vi "Display Info.vi"(7 "Layout ref":refnum<vi>, 8 "error in (no error)":errorcluster, 9 "Modify (F) /Add [T]":bool, 10 "Names in use":string[](array[string]), 11 "NI Card in":refnum<class "NI Card.lvclass">=refnum) -> (0 "error out":errorcluster, 1 "Names in use out":string[](array[string]), 2 "Changes Made?":bool=TRUE, 3 "NI Card out":refnum<class "NI Card.lvclass">)   [LabVIEW 2013, in "NI Card.lvclass"]
uses:
  NI Card.lvclass
  TypeDefs/ColumnAppearCluster.ctl
  TypeDefs/DigitalColumnAppearCluster.ctl
  ColumnVIs/DigitalCol/DigitalCol.lvclass
  ColumnVIs/Column/Column.lvclass
  NI Card.lvclass/NI Card.ctl
panel:
  in  "Set All Analogs":T1={"Column Name"="", "Width"=30, "Bkgd"=[16448250], "Text"=[0]}
  in  "Set All Digitals":T2={"Column Name"="", "Width"=15, "Bkgd"=[1985280, 6618880, 14090026], "Text"=[16448250, 0, 0]}
  in  "Terminal Info":T3={"Trigger terminal"="", "Master\nTrigger Line"=23, "Trigger Mirror"="", "AO Lines"=0, "DO Channel"="", "DO Lines"=0, "AI Pause Line"="", "AI Sample Rate"=0.0, "AI Lines"=0}
  in  "Analog Input Channels":T4(array[cluster])
  in  "Analog Output Channels":T5(array[cluster])
  in  "Digital Output Channels":T2[](array[typedef])
  in  "Cancel":bool
  in  "Done":bool
  in  "Device Description":string
  in  "Name":string="ni"
  # "All Selected channels MUST be from same device! Same goes for \"Terminal Info.\""
  # "Trace color currently does nothing."
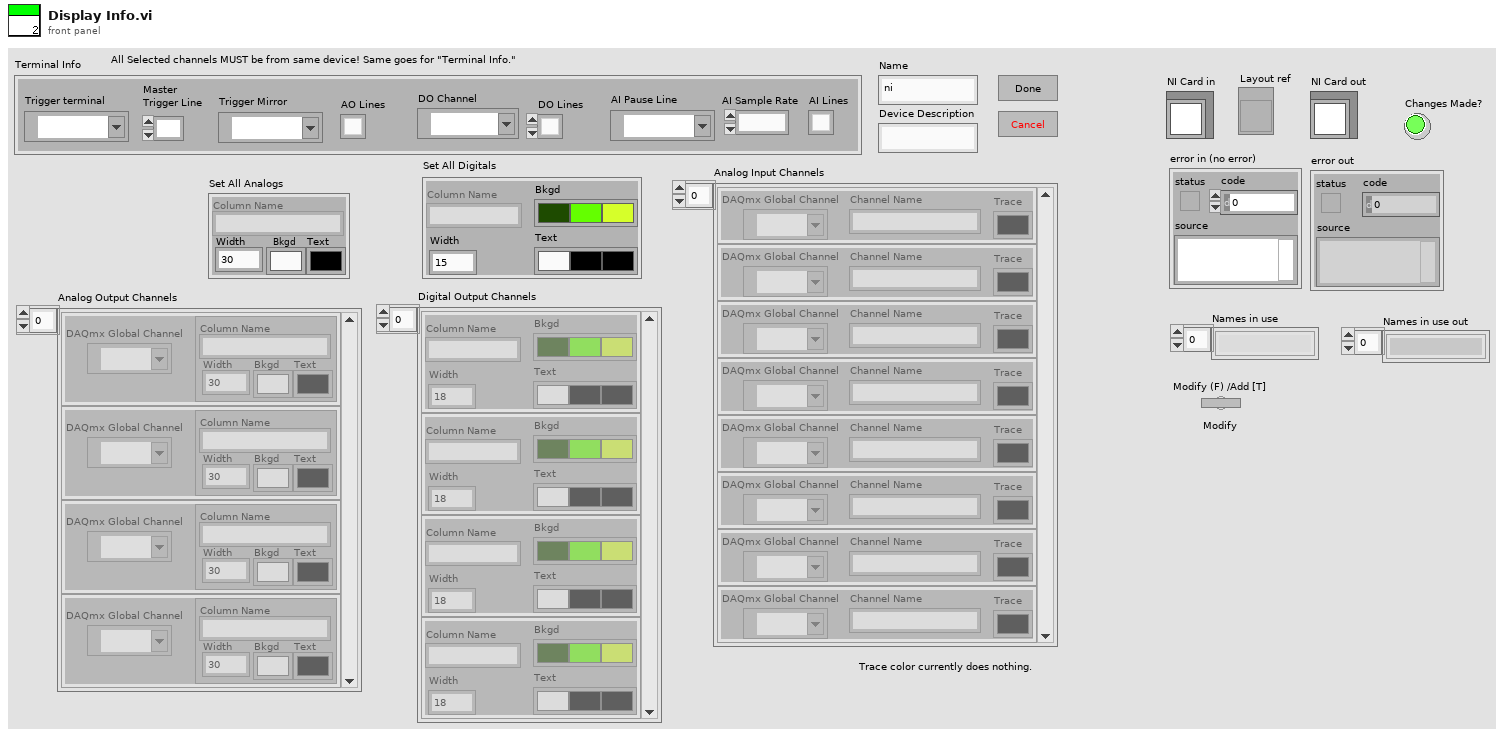
[diagram p1: front panel]
types:
  T1 = typedef "ColumnAppearCluster.ctl" = cluster{"Column Name":string, "Width":u32, "Bkgd":u32[], "Text":u32[]}
  T2 = typedef "DigitalColumnAppearCluster.ctl" = cluster{"Column Name":string, "Width":u32, "Bkgd":u32[], "Text":u32[]}
  T3 = cluster{"Trigger terminal":tag, "Master\nTrigger Line":u16, "Trigger Mirror":tag, "AO Lines":i32, "DO Channel":refnum<k21>, "DO Lines":i32, "AI Pause Line":tag, "AI Sample Rate":dbl, "AI Lines":i32}
  T4 = cluster{"DAQmx Global Channel":refnum<k21>, "Channel Name":string, "Trace":u32[]}[]
  T5 = cluster{"Column Appearance":T1, "DAQmx Global Channel":refnum<k21>}[]
  T6 = cluster{"AI Pause Line":tag, "AI Sample Rate":dbl, "Trigger terminal":tag, "DO Channel":refnum<k21>, "Trigger Mirror":tag}
  T7 = cluster{"DAQmx Global Channel":refnum<k21>, "String":string}[]
  T8 = cluster{"DAQmx Global Channel":refnum<k21>, "Channel Name":string, "Trace":u32[]}
  T9 = cluster{"Column Appearance":T1, "DAQmx Global Channel":refnum<k21>}
  T10 = cluster{"DAQmx Global Channel":refnum<k21>, "Column Name":string}
  T11 = cluster{"DAQmx Global Channel":refnum<k21>, "Channel Name":string}
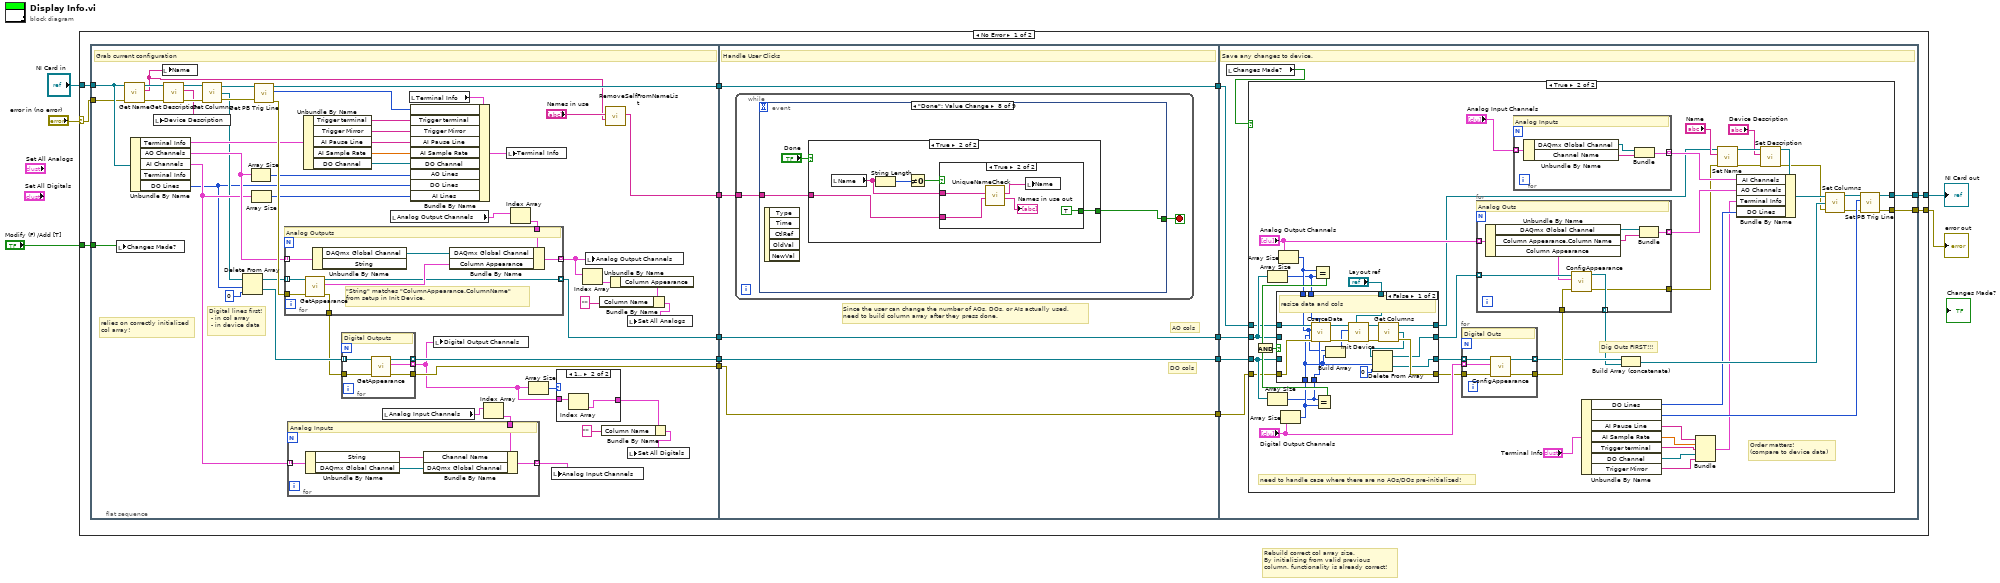
[diagram p0: block diagram]
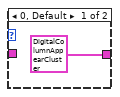
[diagram p2: hidden frame]
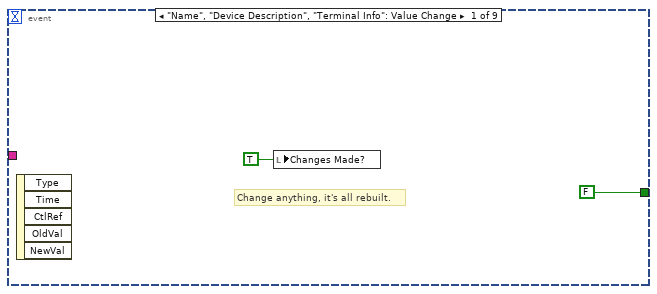
[diagram p3: hidden frame]
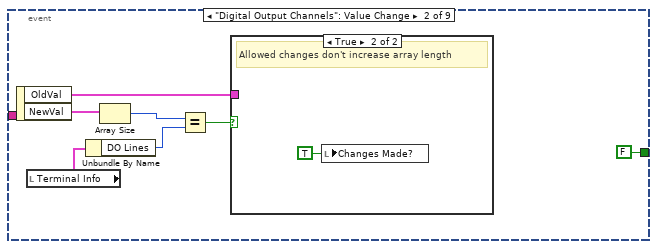
[diagram p4: hidden frame]
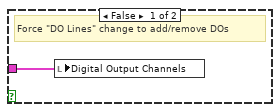
[diagram p5: hidden frame]
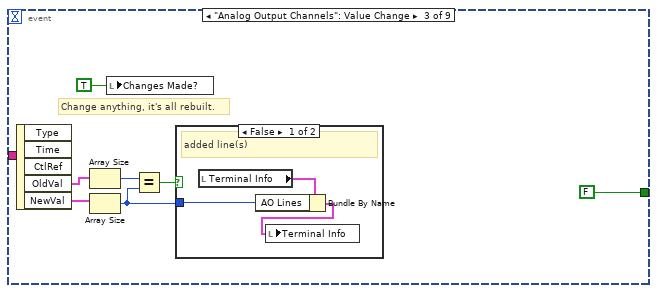
[diagram p6: hidden frame]
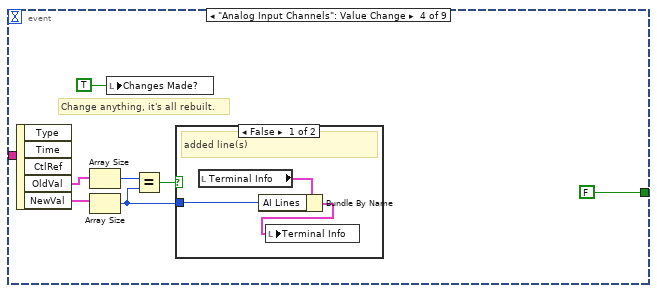
[diagram p8: hidden frame]
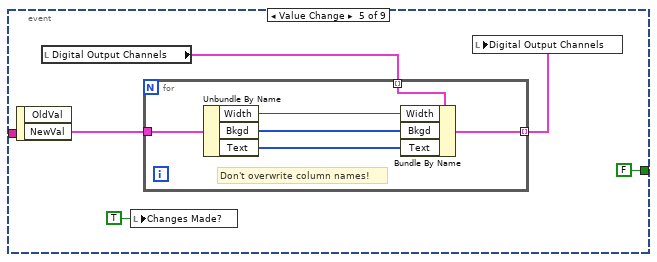
[diagram p10: hidden frame]
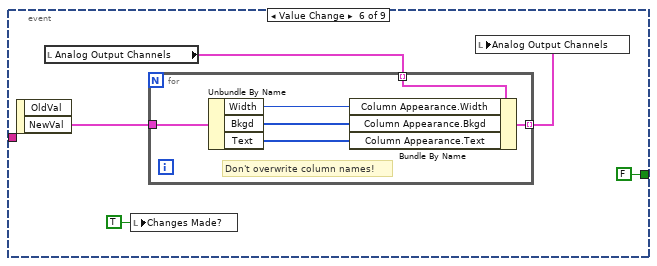
[diagram p11: hidden frame]
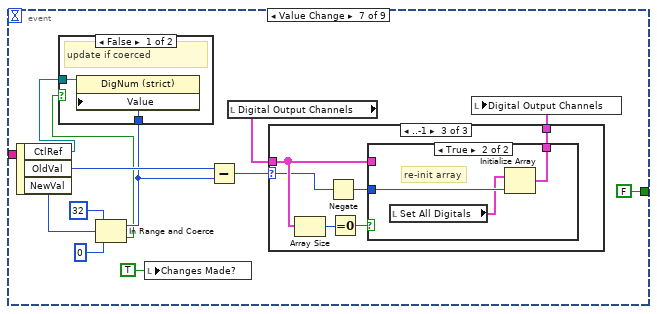
[diagram p12: hidden frame]
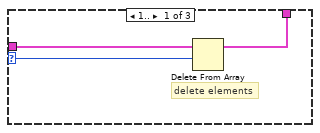
[diagram p14: hidden frame]
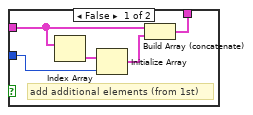
[diagram p16: hidden frame]
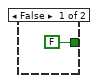
[diagram p17: hidden frame]
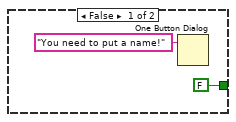
[diagram p18: hidden frame]
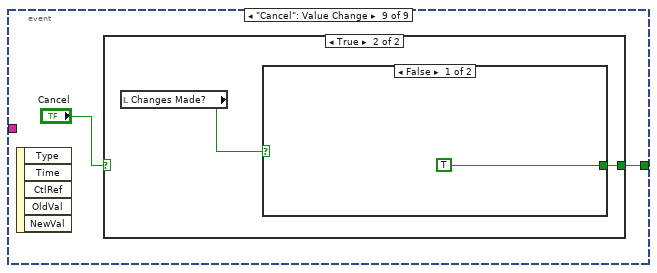
[diagram p19: hidden frame]
diagram:
  # "Rebuild correct col array size.\nBy initializing from valid previous\ncolumn, functionality is already correct!"
  n1 = case shown="No Error" "error in (no error)" {
    selector: "error in (no error)" -> [w16 w308]
    tunnel: "NI Card in" -> [w19 w309]
    tunnel: [w9 w309] -> w3
    tunnel: [w8 w308] -> w2
    tunnel: "Modify (F) /Add [T]" -> [w7 _]
    frame No Error {
      n2 = flat-sequence {
        tunnel: w19 -> [w69]
        tunnel: [w64] -> w18
        tunnel: w16 -> [w43]
        tunnel: [w42] -> w15
        tunnel: [w41] -> w14
        tunnel: [w40] -> w13
        tunnel: w7 -> [w23]
        tunnel: [w20] -> w6
        tunnel: w18 -> [w98]
        tunnel: [w98] -> w17
        tunnel: w15 -> [w95]
        tunnel: w14 -> [w96]
        tunnel: w13 -> [w97]
        tunnel: [w97] -> w12
        tunnel: [w96] -> w11
        tunnel: [w95] -> w10
        tunnel: w6 -> [w94]
        tunnel: w17 -> [w216]
        tunnel: w12 -> [w218]
        tunnel: w11 -> [w217]
        tunnel: w10 -> [w213]
        tunnel: [w215] -> w9
        tunnel: [w214] -> w8
        frame #0 {
          # "relies on correctly initialized\ncol array!"
          # "Digital lines first!\n - in col array\n - in device data"
          # "Grab current configuration"
          n3 = local write "Changes Made?"(w23) -> ()
          n4 = call-dynamic "Get Name.vi"("error in (no error)"=w43, "Device in"=w69) -> ("error out"=w68:errorcluster, "Name"=w21:string, "Device out"=w70:refnum<class "NI Card.lvclass">)  [unwired: 7 in]
          n5 = Unbundle By Name(w69) -> ("Terminal Info"=w57:T6, "AO Channels"=w53:T7, "AI Channels"=w52:T7, "DO Lines"=w32:i32)  [unwired: 1 out]
          n6 = local write "Name"(w21) -> ()
          n7 = call-dynamic "Get Description.vi"("error in (no error)"=w68, "Device in"=w70) -> ("error out"=w66:errorcluster, "Device Description"=w51:string, "Device out"=w67:refnum<class "NI Card.lvclass">)  [unwired: 7 in]
          n8 = local write "Device Description"(w51) -> ()
          n9 = call-dynamic "Get Columns.vi"("Device in"=w67, "error in (no error)"=w66) -> ("Device out"=w65:refnum<class "NI Card.lvclass">, "Columns"=w50:refnum<class "Column.lvclass">[], "error out"=w63:errorcluster)
          n10 = Delete From Array(array=w50, length=w32, index=0) -> (deleted portion=w47:refnum<class "Column.lvclass">[], array with subset deleted=w48:refnum<class "Column.lvclass">[])
          n11 = Array Size(array=w53) -> (size(s)=w55:i32)
          n12 = Array Size(array=w52) -> (size(s)=w54:i32)
          n13 = call-dynamic "Get PB Trig Line.vi"("error in (no error)"=w63, "Device in"=w65) -> ("error out"=w71:errorcluster, "PB Trigger Line"=w45:u16, "Device out"=w64:refnum<class "NI Card.lvclass">)  [unwired: 7 in]
          n14 = Unbundle By Name(w57) -> ("Trigger terminal"=w61:tag, "Trigger Mirror"=w62:tag, "AI Pause Line"=w60:tag, "AI Sample Rate"=w59:dbl, "DO Channel"=w58:refnum<k21>)
          n15 = local read "Analog Input Channels"() -> (w36:T4)
          n16 = local read "Analog Output Channels"() -> (w38:T5)
          n17 = local read "Terminal Info"() -> (w39:T3)
          n18 = Bundle By Name(cluster=w39, "Master\nTrigger Line"=w45, "Trigger terminal"=w61, "Trigger Mirror"=w62, "AI Pause Line"=w60, "AI Sample Rate"=w59, "DO Channel"=w58, "AO Lines"=w55, "DO Lines"=w32, "AI Lines"=w54) -> (w56:T3)
          n19 = Index Array(array=w36) -> (element=w35:T8)  [unwired: 1 in]
          n20 = for {
            tunnel: w52 -> [w84] mode=indexing
            tunnel: w35 -> [w83]
            tunnel: [w80] -> w46 mode=indexing
            # "Analog Inputs"
            n21 = Unbundle By Name(w84) -> ("String"=w82:string, "DAQmx Global Channel"=w81:refnum<k21>)
            n22 = Bundle By Name(cluster=w83, "Channel Name"=w82, "DAQmx Global Channel"=w81) -> (w80:T8)
          }
          n23 = local write "Terminal Info"(w56) -> ()
          n24 = Index Array(array=w38) -> (element=w37:T9)  [unwired: 1 in]
          n25 = for {
            tunnel: w53 -> [w93] mode=indexing
            tunnel: w48 -> [w89] mode=indexing
            tunnel: [w90] -> w34 mode=indexing
            tunnel: w71 -> [w88]
            tunnel: [w87] -> w44
            tunnel: [w86] -> w40 mode=indexing
            tunnel: w37 -> [w85]
            # "\"String\" matches \"ColumnAppearance.ColumnName\"\nfrom setup in Init Device."
            # "Analog Outputs"
            n26 = call "GetAppearance.vi"("error in (no error)"=w88, "Column in"=w89) -> ("error out"=w87:errorcluster, "Column Appearance"=w91:T1, "Column out"=w86:refnum<class "Column.lvclass">)  [unwired: 7 in]
            n27 = Unbundle By Name(w93) -> ("DAQmx Global Channel"=w92:refnum<k21>)  [unwired: 1 out]
            n28 = Bundle By Name(cluster=w85, "DAQmx Global Channel"=w92, "Column Appearance"=w91) -> (w90:T9)
          }
          n29 = for {
            tunnel: w47 -> [w79] mode=indexing
            tunnel: [w78] -> w31 mode=indexing
            tunnel: w44 -> [w77]
            tunnel: [w76] -> w42
            tunnel: [w75] -> w41 mode=indexing
            # "Digital Outputs"
            n30 = call "GetAppearance.vi"("error in (no error)"=w77, "Column in"=w79) -> ("error out"=w76:errorcluster, "Column Appearance"=w78:T1, "Column out"=w75:refnum<class "Column.lvclass">)  [unwired: 7 in]
          }
          n31 = local write "Digital Output Channels"(w31) -> ()
          n32 = Array Size(array=w31) -> (size(s)=w30:i32)
          n33 = local write "Analog Input Channels"(w46) -> ()
          n34 = case shown="1.." w30 {
            tunnel: w31 -> [_ w74]
            tunnel: [T2 {"Column Name"="", "Width"=15, "Bkgd"=[1985280, 6618880, 14090026], "Text"=[16448250, 0, 0]} ("Set All Digitals") w73] -> w25
            frame 0, Default {
            }
            frame 1.. {
              n35 = Index Array(array=w74) -> (element=w73:T1)  [unwired: 1 in]
            }
          }
          n36 = Index Array(array=w34) -> (element=w33:T9)  [unwired: 1 in]
          n37 = local write "Analog Output Channels"(w34) -> ()
          n38 = Bundle By Name(cluster=w25, "Column Name"="") -> (w24:T1)
          n39 = call "RemoveSelfFromNameList.vi"("self Name"=w21, "Names in use"="Names in use") -> ("Reserved Names"=w20:string[])  [unwired: 9 in]
          n40 = Unbundle By Name(w33) -> ("Column Appearance"=w29:T1)
          n41 = Bundle By Name(cluster=w29, "Column Name"="") -> (w27:T1)
          n42 = local write "Set All Analogs"(w27) -> ()
          n43 = local write "Set All Digitals"(w24) -> ()
        }
        frame #1 {
          # "DO cols"
          # "AO cols"
          # "Since the user can change the number of AOs, DOs, or AIs actually used, \nneed to build column array after they press done."
          # "Handle User Clicks"
          n44 = while {
            tunnel: w94 -> [w99]
            stop <- w100 stop-if-true
            n45 = event shown="[7] \"Done\": Value Change" {
              selector: _ -> [_ _ _ _ _ _ _ _ _]
              dyn-events: _ -> [_ _ _ _ _ _ _ _ _]
              timeout: _ -> [_ _ _ _ _ _ _ _ _]
              tunnel: [FALSE ("T button?") FALSE ("T button?") FALSE ("T button?") FALSE ("T button?") FALSE ("T button?") FALSE ("T button?") FALSE ("T button?") w187 w202] -> w100
              tunnel: w99 -> [_ _ _ _ _ _ _ w186 _]
              event "Name", "Device Description", "Terminal Info": Value Change {
                # "Change anything, it's all rebuilt."
                n46 = event-data() -> ()  [unwired: 1 in, 5 out]
                n47 = local write "Changes Made?"(TRUE) -> ()
              }
              event "Digital Output Channels": Value Change {
                n48 = event-data() -> ("OldVal"=w104:T2[], "NewVal"=w109:T2[])  [unwired: 1 in]
                n49 = local read "Terminal Info"() -> (w108:T3)
                n50 = Unbundle By Name(w108) -> ("DO Lines"=w106:i32)
                n51 = Array Size(array=w109) -> (size(s)=w107:i32)
                n52 = Equal?(x=w107, y=w106) -> (x = y?=w105:bool)
                n53 = case shown="True" w105 {
                  tunnel: w104 -> [w110 _]
                  frame False {
                    # "Force \"DO Lines\" change to add/remove DOs"
                    n54 = local write "Digital Output Channels"(w110) -> ()
                  }
                  frame True {
                    # "Allowed changes don't increase array length"
                    n55 = local write "Changes Made?"(TRUE ("Changes Made?")) -> ()
                  }
                }
              }
              event "Analog Output Channels": Value Change {
                # "Change anything, it's all rebuilt."
                n56 = event-data() -> ("OldVal"=w115:T5, "NewVal"=w116:T5)  [unwired: 1 in, 3 out]
                n57 = Array Size(array=w115) -> (size(s)=w114:i32)
                n58 = Array Size(array=w116) -> (size(s)=w112:i32)
                n59 = local write "Changes Made?"(TRUE) -> ()
                n60 = Equal?(x=w114, y=w112) -> (x = y?=w113:bool)
                n61 = case shown="False" w113 {
                  tunnel: w112 -> [w120 _]
                  frame False {
                    # "added line(s)"
                    n62 = local read "Terminal Info"() -> (w121:T3)
                    n63 = Bundle By Name(cluster=w121, "AO Lines"=w120) -> (w119:T3)
                    n64 = local write "Terminal Info"(w119) -> ()
                  }
                  frame True {
                    # "same number of lines"
                  }
                }
              }
              event "Analog Input Channels": Value Change {
                # "Change anything, it's all rebuilt."
                n65 = event-data() -> ("OldVal"=w125:T4, "NewVal"=w126:T4)  [unwired: 1 in, 3 out]
                n66 = Array Size(array=w125) -> (size(s)=w124:i32)
                n67 = Array Size(array=w126) -> (size(s)=w122:i32)
                n68 = local write "Changes Made?"(TRUE) -> ()
                n69 = Equal?(x=w124, y=w122) -> (x = y?=w123:bool)
                n70 = case shown="False" w123 {
                  tunnel: w122 -> [w130 _]
                  frame False {
                    # "added line(s)"
                    n71 = local read "Terminal Info"() -> (w131:T3)
                    n72 = Bundle By Name(cluster=w131, "AI Lines"=w130) -> (w129:T3)
                    n73 = local write "Terminal Info"(w129) -> ()
                  }
                  frame True {
                    # "same number of lines"
                  }
                }
              }
              event Value Change {
                n74 = event-data() -> ("NewVal"=w132:T2)  [unwired: 1 in, 1 out]
                n75 = local read "Digital Output Channels"() -> (w134:T2[])
                n76 = local write "Changes Made?"(TRUE ("Changes Made?")) -> ()
                n77 = for {
                  tunnel: w134 -> [w142] mode=indexing
                  tunnel: [w141] -> w133 mode=indexing
                  tunnel: w132 -> [w140]
                  # "Don't overwrite column names!"
                  n78 = Unbundle By Name(w140) -> ("Width"=w139:u32, "Bkgd"=w138:u32[], "Text"=w137:u32[])
                  n79 = Bundle By Name(cluster=w142, "Width"=w139, "Bkgd"=w138, "Text"=w137) -> (w141:T2)
                }
                n80 = local write "Digital Output Channels"(w133) -> ()
              }
              event Value Change {
                n81 = event-data() -> ("NewVal"=w143:T1)  [unwired: 1 in, 1 out]
                n82 = local read "Analog Output Channels"() -> (w145:T5)
                n83 = local write "Changes Made?"(TRUE ("Changes Made?")) -> ()
                n84 = for {
                  tunnel: w145 -> [w153] mode=indexing
                  tunnel: [w152] -> w144 mode=indexing
                  tunnel: w143 -> [w151]
                  # "Don't overwrite column names!"
                  n85 = Unbundle By Name(w151) -> ("Width"=w150:u32, "Bkgd"=w149:u32[], "Text"=w148:u32[])
                  n86 = Bundle By Name(cluster=w153, "Column Appearance.Width"=w150, "Column Appearance.Bkgd"=w149, "Column Appearance.Text"=w148) -> (w152:T9)
                }
                n87 = local write "Analog Output Channels"(w144) -> ()
              }
              event "Terminal Info.DO Lines": Value Change {
                n88 = event-data() -> ("CtlRef"=w156:refnum<vi>, "OldVal"=w165:i32, "NewVal"=w157:i32)  [unwired: 1 in]
                n89 = In Range and Coerce(upper limit=32 ("y"), x=w157, lower limit=0) -> (coerced(x)=w155:i32, In Range?=w154:bool)
                n90 = case shown="False" w154 {
                  tunnel: w156 -> [w167 _]
                  tunnel: w155 -> [w166 _]
                  frame False {
                    # "update if coerced"
                    n91 = property class="DigNum (strict)"(reference=w167, "Value"=w166) -> ()  [unwired: 1 in, 2 out]
                  }
                  frame True {
                  }
                }
                n92 = local write "Changes Made?"(TRUE ("Changes Made?")) -> ()
                n93 = Subtract(x=w165, y=w155) -> (x-y=w162:i32)
                n94 = local read "Digital Output Channels"() -> (w161:T2[])
                n95 = case shown="..-1" w162 {
                  selector: w162 -> [w170 _ w172]
                  tunnel: w161 -> [w169 w171 w176]
                  tunnel: [w168 w171 w177] -> w160
                  frame 1.. {
                    # "delete elements"
                    n96 = Delete From Array(array=w169, length=w170) -> (array with subset deleted=w168:T2[])  [unwired: 1 in, 1 out]
                  }
                  frame 0, Default {
                  }
                  frame ..-1 {
                    n97 = Array Size(array=w176) -> (size(s)=w175:i32)
                    n98 = Negate(x=w172) -> (-x=w173:i32)
                    n99 = Equal To 0?(x=w175) -> (x = 0?=w174:bool)
                    n100 = case shown="True" w174 {
                      tunnel: [w182 w184] -> w177
                      tunnel: w173 -> [w179 w185]
                      tunnel: w176 -> [w181 _]
                      frame False {
                        # "add additional elements (from 1st)"
                        n101 = Index Array(array=w181) -> (element=w180:T2)  [unwired: 1 in]
                        n102 = Initialize Array(w180, w179) -> (w178:T2[])
                        n103 = Build Array (concatenate)(w181, w178) -> (w182:T2[])
                      }
                      frame True {
                        # "re-init array"
                        n104 = local read "Set All Digitals"() -> (w183:T2)
                        n105 = Initialize Array(w183, w185) -> (w184:T2[])
                      }
                    }
                  }
                }
                n106 = local write "Digital Output Channels"(w160) -> ()
              }
              event "Done": Value Change {
                n107 = event-data() -> ()  [unwired: 1 in, 5 out]
                n108 = case shown="True" "Done" {
                  tunnel: [FALSE w192] -> w187
                  tunnel: w186 -> [_ w190]
                  frame False {
                  }
                  frame True {
                    n109 = local read "Name"() -> (w191:string)
                    n110 = String Length(string=w191) -> (length=w194:i32)
                    n111 = Not Equal To 0?(x=w194) -> (x != 0?=w193:bool)
                    n112 = case shown="True" w193 {
                      tunnel: [FALSE TRUE] -> w192
                      tunnel: w191 -> [_ w200]
                      tunnel: w190 -> [_ w198]
                      frame False {
                        n113 = One Button Dialog(message="You need to put a name!") -> ()  [unwired: 1 in, 1 out]
                      }
                      frame True {
                        n114 = call "UniqueNameCheck.vi"("Names in use"=w198, "Device Name"=w200) -> ("Names in use out"=→"Names in use out":string[], "Unique name"=w199:string)  [unwired: 8 in]
                        n115 = local write "Name"(w199) -> ()
                      }
                    }
                  }
                }
              }
              event "Cancel": Value Change {
                n116 = event-data() -> ()  [unwired: 1 in, 5 out]
                n117 = case shown="True" "Cancel" {
                  selector: "Cancel" -> [w204 _]
                  tunnel: [w204 w206] -> w202
                  frame False {
                  }
                  frame True {
                    n118 = local read "Changes Made?"() -> (w205:bool)
                    n119 = case shown="False" w205 {
                      tunnel: [TRUE w209] -> w206
                      frame False {
                      }
                      frame True {
                        n120 = Two Button Dialog(message="Are you sure you want to cancel without saving changes?", 1:"No", 2:"Yes") -> (T button?=w209:bool)
                        n121 = Not(x=w209) -> (.not. x?=w208:bool)
                        n122 = local write "Changes Made?"(w208) -> ()
                      }
                    }
                  }
                }
              }
            }
          }
        }
        frame #2 {
          # "Save any changes to device."
          n123 = local read "Changes Made?"() -> (w219:bool)
          n124 = case shown="True" w219 {
            tunnel: w218 -> [_ w234]
            tunnel: w217 -> [_ w233]
            tunnel: w216 -> [w221 w224]
            tunnel: [w221 w239] -> w215
            tunnel: [w220 w238] -> w214
            tunnel: w213 -> [w220 w226]
            frame False {
            }
            frame True {
              # "need to handle case where there are no AOs/DOs pre-initialized!"
              # "Order matters!\n(compare to device data)"
              # "Dig Outs FIRST!!!"
              n125 = Array Size(array=w234) -> (size(s)=w227:i32)
              n126 = Array Size(array=w233) -> (size(s)=w228:i32)
              n127 = Array Size(array="Analog Output Channels") -> (size(s)=w229:i32)
              n128 = Array Size(array="Digital Output Channels") -> (size(s)=w230:i32)
              n129 = Equal?(x=w229, y=w227) -> (x = y?=w237:bool)
              n130 = Equal?(x=w228, y=w230) -> (x = y?=w236:bool)
              n131 = And(x=w237, y=w236) -> (x .and. y?=w235:bool)
              n132 = case shown="False" w235 {
                tunnel: w234 -> [_ w289]
                tunnel: w233 -> [_ w288]
                tunnel: [w269 w289] -> w231
                tunnel: [w268 w288] -> w232
                tunnel: w230 -> [w271 _]
                tunnel: w229 -> [w279 _]
                tunnel: w228 -> [w284 _]
                tunnel: w227 -> [w283 _]
                tunnel: w226 -> [w282 w287]
                tunnel: [w273 w287] -> w225
                tunnel: w224 -> [w285 w286]
                tunnel: [w274 w286] -> w223
                tunnel: "Layout ref" -> [w277 _]
                frame False {
                  # "resize data and cols"
                  n133 = call "CoerceData.vi"("Old DO sizes"=w284, "Old AO sizes"=w283, "error in (no error)"=w282, "New DO sizes"=w271, "New AO sizes"=w279, "NI Card in"=w285) -> ("error out"=w280:errorcluster, "NI Card out"=w281:refnum<class "NI Card.lvclass">)  [unwired: 4 in]
                  n134 = Build Array(w279, w271) -> (w278:i32[])
                  n135 = call-dynamic "Init Device.vi"("Layout Ref"=w277, "error in (no error)"=w280, "Chan# Array"=w278, "NI Card in"=w281) -> ("error out"=w276:errorcluster, "NI Card out"=w275:refnum<class "NI Card.lvclass">)  [unwired: 6 in]
                  n136 = call-dynamic "Get Columns.vi"("Device in"=w275, "error in (no error)"=w276) -> ("Device out"=w274:refnum<class "NI Card.lvclass">, "Columns"=w272:refnum<class "Column.lvclass">[], "error out"=w273:errorcluster)
                  n137 = Delete From Array(array=w272, length=w271, index=0) -> (deleted portion=w268:refnum<class "Column.lvclass">[], array with subset deleted=w269:refnum<class "Column.lvclass">[])
                }
                frame True {
                  # "# AOs/DOs cols OK"
                }
              }
              n138 = for {
                tunnel: w232 -> [w294] mode=indexing
                tunnel: [w293] -> w256 mode=indexing
                tunnel: "Digital Output Channels" -> [w292] mode=indexing
                tunnel: w225 -> [w291]
                tunnel: [w290] -> w258
                # "Digital Outs"
                n139 = call "ConfigAppearance.vi"("error in (no error)"=w291, "Column Appearance"=w292, "Column in"=w294) -> ("error out"=w290:errorcluster, "Column out"=w293:refnum<class "Column.lvclass">)  [unwired: 7 in]
              }
              n140 = for {
                tunnel: "Analog Output Channels" -> [w302] mode=indexing
                tunnel: w231 -> [w303] mode=indexing
                tunnel: [w298] -> w252 mode=indexing
                tunnel: [w297] -> w255 mode=indexing
                tunnel: w258 -> [w296]
                tunnel: [w295] -> w244
                # "Analog Outs"
                n141 = Unbundle By Name(w302) -> ("DAQmx Global Channel"=w300:refnum<k21>, "Column Appearance.Column Name"=w299:string, "Column Appearance"=w301:T1)
                n142 = call "ConfigAppearance.vi"("error in (no error)"=w296, "Column Appearance"=w301, "Column in"=w303) -> ("error out"=w295:errorcluster, "Column out"=w297:refnum<class "Column.lvclass">)  [unwired: 7 in]
                n143 = Bundle("DAQmx Global Channel"=w300, "Column Name"=w299) -> (w298:T10)  [unwired: 1 in]
              }
              n144 = for {
                tunnel: "Analog Input Channels" -> [w307] mode=indexing
                tunnel: [w306] -> w253 mode=indexing
                # "Analog Inputs"
                n145 = Unbundle By Name(w307) -> ("DAQmx Global Channel"=w304:refnum<k21>, "Channel Name"=w305:string)
                n146 = Bundle("DAQmx Global Channel"=w304, "Channel Name"=w305) -> (w306:T11)  [unwired: 1 in]
              }
              n147 = Unbundle By Name("Terminal Info") -> ("DO Lines"=w247:i32, "Master\nTrigger Line"=w246:u16, "AI Pause Line"=w265:tag, "AI Sample Rate"=w261:dbl, "Trigger terminal"=w264:tag, "DO Channel"=w263:refnum<k21>, "Trigger Mirror"=w262:tag)
              n148 = Build Array (concatenate)(w256, w255) -> (w249:refnum<class "Column.lvclass">[])
              n149 = Bundle("AI Pause Line"=w265, "AI Sample Rate"=w261, "Trigger terminal"=w264, "DO Channel"=w263, "Trigger Mirror"=w262) -> (w240:T6)  [unwired: 1 in]
              n150 = call-dynamic "Set Name.vi"("error in (no error)"=w244, "Name"="Name", "Device in"=w223) -> ("error out"=w250:errorcluster, "Device out"=w267:refnum<class "NI Card.lvclass">)  [unwired: 7 in]
              n151 = call-dynamic "Set Description.vi"("error in (no error)"=w250, "Device Description"="Device Description", "Device in"=w267) -> ("error out"=w243:errorcluster, "Device out"=w245:refnum<class "NI Card.lvclass">)  [unwired: 7 in]
              n152 = Bundle By Name(cluster=w245, "AI Channels"=w253, "AO Channels"=w252, "Terminal Info"=w240, "DO Lines"=w247) -> (w251:refnum<class "NI Card.lvclass">)
              n153 = call-dynamic "Set Columns.vi"("error in (no error)"=w243, "Columns"=w249, "NI Card in"=w251) -> ("error out"=w241:errorcluster, "NI Card out"=w242:refnum<class "NI Card.lvclass">)  [unwired: 1 in]
              n154 = call-dynamic "Set PB Trig Line.vi"("error in (no error)"=w241, "PB Trigger Line"=w246, "Device in"=w242) -> ("error out"=w238:errorcluster, "Device out"=w239:refnum<class "NI Card.lvclass">)  [unwired: 7 in]
            }
          }
        }
      }
    }
    frame Error {
      (unwired) FALSE
    }
  }
  "error out" <- w2
  "NI Card out" <- w3
